vi "Build Missing Tree Error.vi"(0 "Unique ID":string, 11 "Error In":errorcluster) -> (15 "Error Out":errorcluster)   [LabVIEW 2017, in "Tree API.lvlib" / "Tree.lvclass"]
uses:
  Tree.lvclass
  <vilib>/ErrorRing/Error Ring.xnode
  <vilib>/Utility/error.llb/Error Cluster From Error Code.vi
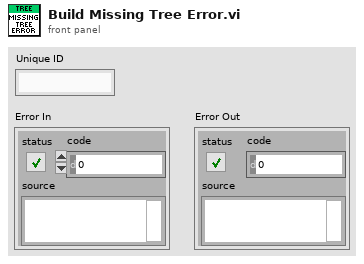
[diagram p1: front panel]
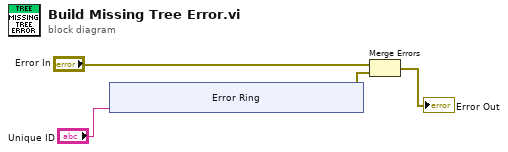
[diagram p0: block diagram]
diagram:
  n1 = xnode "Error Ring"("参数 0"="Unique ID") -> ("错误输出"=w2:errorcluster)
  n2 = Merge Errors("Error In", w2) -> (→"Error Out":errorcluster)
